vi "Stop Core.vi"(10 "final error code":i32, 11 "UI Actor in":refnum<class "UI Actor.lvclass">) -> (3 "UI Actor out":refnum<class "UI Actor.lvclass">)   [LabVIEW 2020, in "UI Actor.lvlib" / "UI Actor.lvclass"]
doc: "<p>(<strong>Filename</strong>: <span class=\"dnl\">Actor Framework.lvlib:Actor.lvclass:Stop Core.vi</span>)</p>\n<p>Defines what the actor does before it stops. Use the <strong>final error code</strong> input to determine whether the actor shut down in response to an error.</p>\n<p>By default, this method passes the Stop message along to all <a href=\"nihelplauncher://docs/csh?context=lvcore_lvcomm_af_launch_nested_actor\">auto-stop nested actors</a>. A descendant class may override this method to define additional behavior, such as shutting down any processes the actor initiated in its override of the <a href=\"nihelplauncher://docs/csh?context=lvcore_lvcomm_af_actor_core\">Actor Core</a> method.</p>"
uses:
  UI Actor.lvclass
  UI Actor.lvclass/UI Actor.ctl
  <vilib>/MGI/Panel Manager/Panel Actor/Panel Actor/Panel Actor.lvclass
  PDO Grid/PDO Grid.lvclass
  Electronic Datasheet/Electronic Datasheet.lvclass
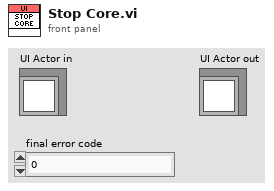
[diagram p1: front panel]
types:
  T1 = map{path, refnum<class "Electronic Datasheet.lvclass">}
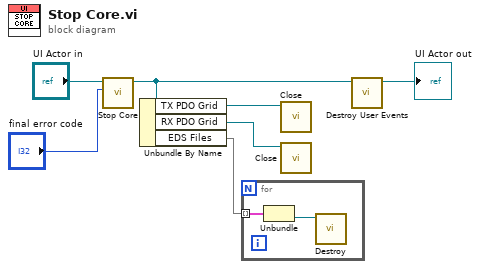
[diagram p0: block diagram]
diagram:
  n1 = call-parent "Stop Core.vi"("final error code"="final error code", "Actor in"="UI Actor in") -> ("Actor out"=w5:refnum<class "UI Actor.lvclass">)  [unwired: 9 in]
  n2 = Unbundle By Name(w5) -> ("TX PDO Grid"=w4:refnum<class "PDO Grid.lvclass">, "RX PDO Grid"=w2:refnum<class "PDO Grid.lvclass">, "EDS Files"=w1:T1)
  n3 = for {
    tunnel: w1 -> [w9] mode=indexing
    n4 = Unbundle(w9) -> ("EDS"=w8:refnum<class "Electronic Datasheet.lvclass">)  [unwired: 1 out]
    n5 = call-dynamic "Destroy.vi"("reference in"=w8) -> ()  [unwired: 9 in, 2 out]
  }
  n6 = call-dynamic "Close.vi"("Sourcegrid in"=w4) -> ()  [unwired: 9 in, 2 out]
  n7 = call-dynamic "Close.vi"("Sourcegrid in"=w2) -> ()  [unwired: 9 in, 2 out]
  n8 = call "Destroy User Events.vi"("UI Actor in"=w5) -> ("UI Actor out"=→"UI Actor out":refnum<class "UI Actor.lvclass">)  [unwired: 10 in]
